vi "Destroy View.vi"(0 "Serial port assistant view in":refnum<class "Serial port assistant view.lvclass">, 11 "error in (no error)":errorcluster) -> (4 "Serial port assistant view out":refnum<class "Serial port assistant view.lvclass">, 15 "error out":errorcluster)   [LabVIEW 2022 SP3, in "Serial port assistant view.lvlib" / "Serial port assistant view.lvclass"]
uses:
  Serial port assistant view.lvclass
  Serial port assistant view.lvclass/Serial port assistant view.ctl
  forced exit--type.ctl
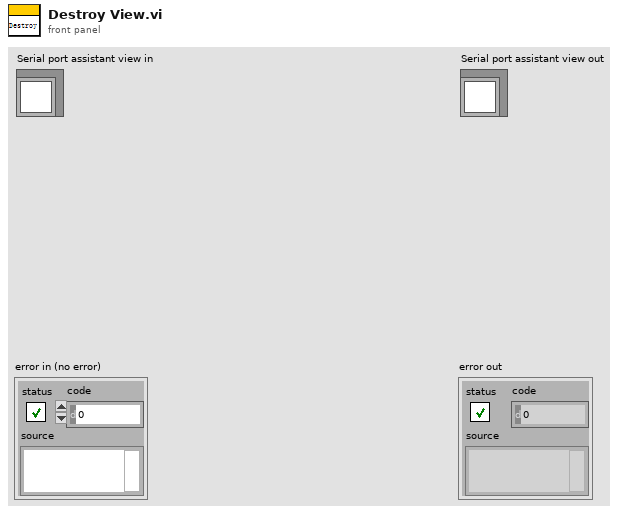
[diagram p1: front panel]
types:
  T1 = enum32{"Bad", "Idle", "Run top level", "Running"}
  T2 = typedef "Serial port assistant view.lvlib/Serial port assistant view.lvclass/forced exit--type.ctl" = cluster{"message":string}
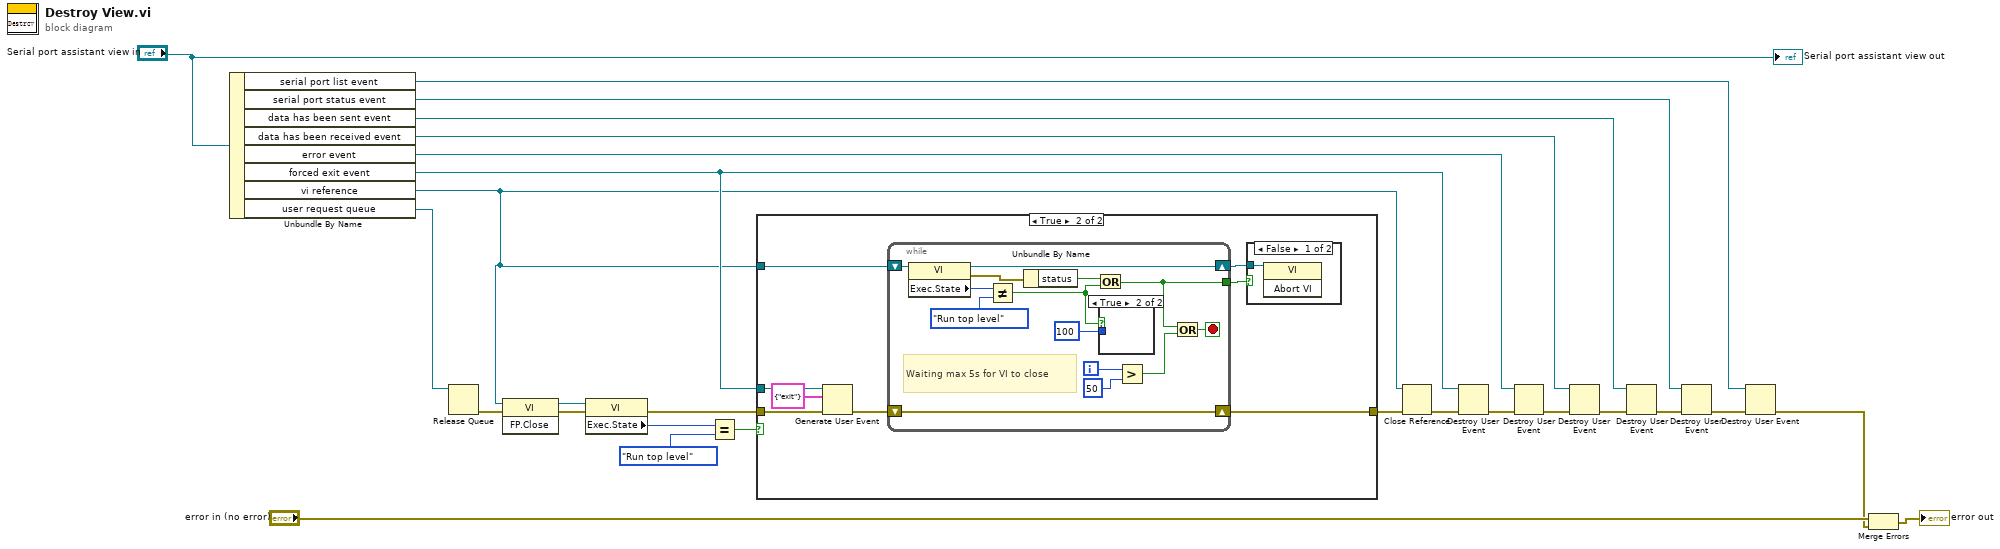
[diagram p0: block diagram]
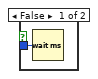
[diagram p4: hidden frame]
diagram:
  n1 = Unbundle By Name("Serial port assistant view in") -> ("serial port list event"=w18:refnum<user-event>, "serial port status event"=w17:refnum<user-event>, "data has been sent event"=w16:refnum<user-event>, "data has been received event"=w15:refnum<user-event>, "error event"=w14:refnum<user-event>, "forced exit event"=w7:refnum<user-event>, "vi reference"=w3:refnum<vi>, "user request queue"=w12:refnum<queue>)
  n2 = Release Queue(queue=w12) -> (error out=w4:errorcluster)  [unwired: 2 in, 2 out]
  n3 = invoke class="VI" method="FP.Close"(reference=w3, error in=w4) -> (reference out=w2:refnum<vi>, error out=w1:errorcluster)  [unwired: 1 in, 1 out]
  n4 = property class="VI"(reference=w2, error in=w1) -> (error out=w8:errorcluster, "Exec.State"=w11:T1)  [unwired: 1 out]
  n5 = Equal?(x=w11, y=T1."Run top level") -> (x = y?=w9:bool)
  n6 = case shown="True" w9 {
    tunnel: w8 -> [w27 w35]
    tunnel: w7 -> [_ w34]
    tunnel: [w27 w29] -> w5
    tunnel: w3 -> [_ w28]
    frame False {
    }
    frame True {
      n7 = Generate User Event(user event=w34, event data cluster=T2 {"message"="exit"} ("event data"), error in=w35) -> (error out=w30:errorcluster)  [unwired: 1 in, 1 out]
      n8 = while {
        tunnel: [w38] -> w31
        shift-right: [w45] -> w29
        shift-left: w30 -> [w45]
        shift-right: [w43] -> w32
        shift-left: w28 -> [w44]
        i -> [w49]
        stop <- w46 stop-if-true
        # "Waiting max 5s for VI to close"
        n9 = property class="VI"(reference=w44) -> (reference out=w43:refnum<vi>, error out=w40:errorcluster, "Exec.State"=w42:T1)  [unwired: 1 in]
        n10 = Not Equal?(x=w42, y=T1."Run top level") -> (x != y?=w37:bool)
        n11 = Unbundle By Name(w40) -> ("status"=w39:bool)
        n12 = Or(x=w39, y=w37) -> (x .or. y?=w38:bool)
        n13 = case shown="True" w37 {
          tunnel: u32 100 ("milliseconds to wait") -> [w51 _]
          frame False {
            n14 = Wait (ms)(milliseconds to wait=w51) -> ()  [unwired: 1 out]
          }
          frame True {
          }
        }
        n15 = Greater?(x=w49, y=50) -> (0:w47:bool)
        n16 = Or(x=w38, y=w47) -> (x .or. y?=w46:bool)
      }
      n17 = case shown="False" w31 {
        tunnel: w32 -> [w36 _]
        frame False {
          n18 = invoke class="VI" method="Abort VI"(reference=w36) -> ()  [unwired: 2 in, 3 out]
        }
        frame True {
        }
      }
    }
  }
  n19 = Close Reference(reference=w3, error in (no error)=w5) -> (error out=w13:errorcluster)
  n20 = Destroy User Event(user event=w7, error in=w13) -> (error out=w25:errorcluster)
  n21 = Destroy User Event(user event=w14, error in=w25) -> (error out=w24:errorcluster)
  n22 = Destroy User Event(user event=w15, error in=w24) -> (error out=w23:errorcluster)
  n23 = Destroy User Event(user event=w16, error in=w23) -> (error out=w20:errorcluster)
  n24 = Destroy User Event(user event=w17, error in=w20) -> (error out=w19:errorcluster)
  n25 = Destroy User Event(user event=w18, error in=w19) -> (error out=w6:errorcluster)
  n26 = Merge Errors("error in (no error)", w6) -> (→"error out":errorcluster)
  "Serial port assistant view out" <- "Serial port assistant view in"
